vi "Read.vi"(0 "Setpoint Array":waveform(dbl)[](array[waveform]), 7 "error in (no error)":errorcluster, 14 "Process_REF":string="Temperature", 15 "physical channels":tag, 17 "Abort":bool) -> (20 "Temperature Graph":waveform(dbl)[](graph), 21 "Thermocouple 1":dbl, 22 "Thermocouple 2":dbl, 23 "Thermocouple 3":dbl, 24 "Thermocouple 4":dbl, 25 "Thermocouple 5":dbl, 27 "error out":errorcluster)   [LabVIEW 2018]
uses:
  <vilib>/DAQmx/read.llb/DAQmx Read (Analog 1D DBL NChan 1Samp).vi
  <vilib>/DAQmx/create/channels.llb/DAQmx Create Channel (AI-Temperature-Thermocouple).vi
  <vilib>/DAQmx/miscellaneous.llb/DAQmx Fill In Error Info.vi
  <vilib>/Waveform/WDTOps.llb/WDT Append Waveforms DBL.vi
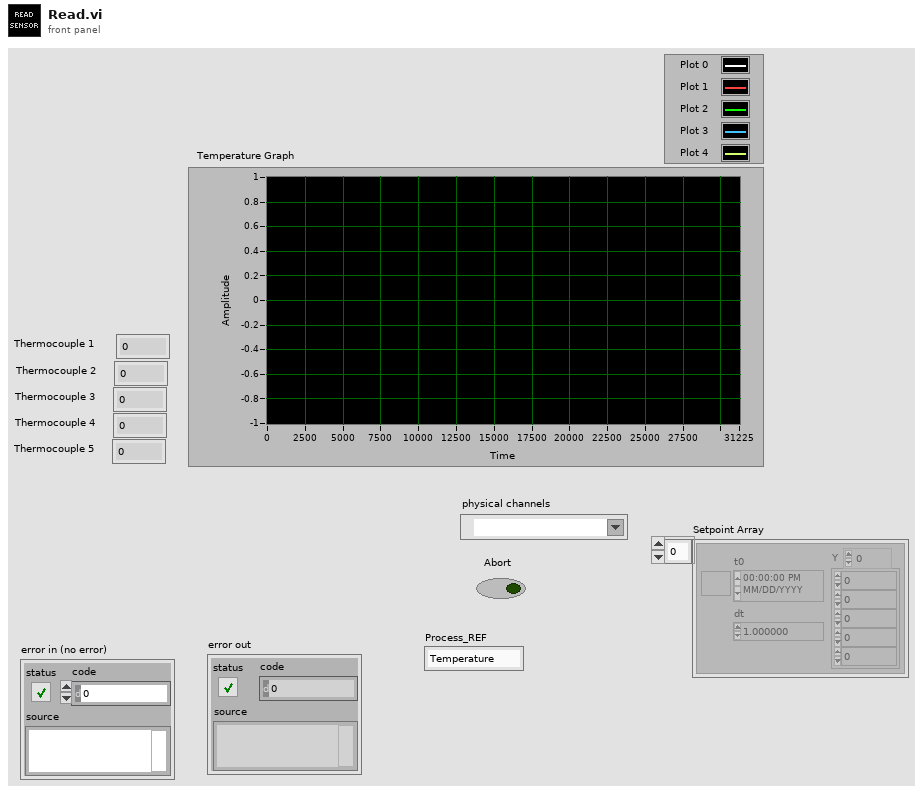
[diagram p1: front panel]
types:
  T1 = cluster{"data[0]":dbl, "data[1]":dbl, "data[2]":dbl, "data[3]":dbl, "data[4]":dbl}
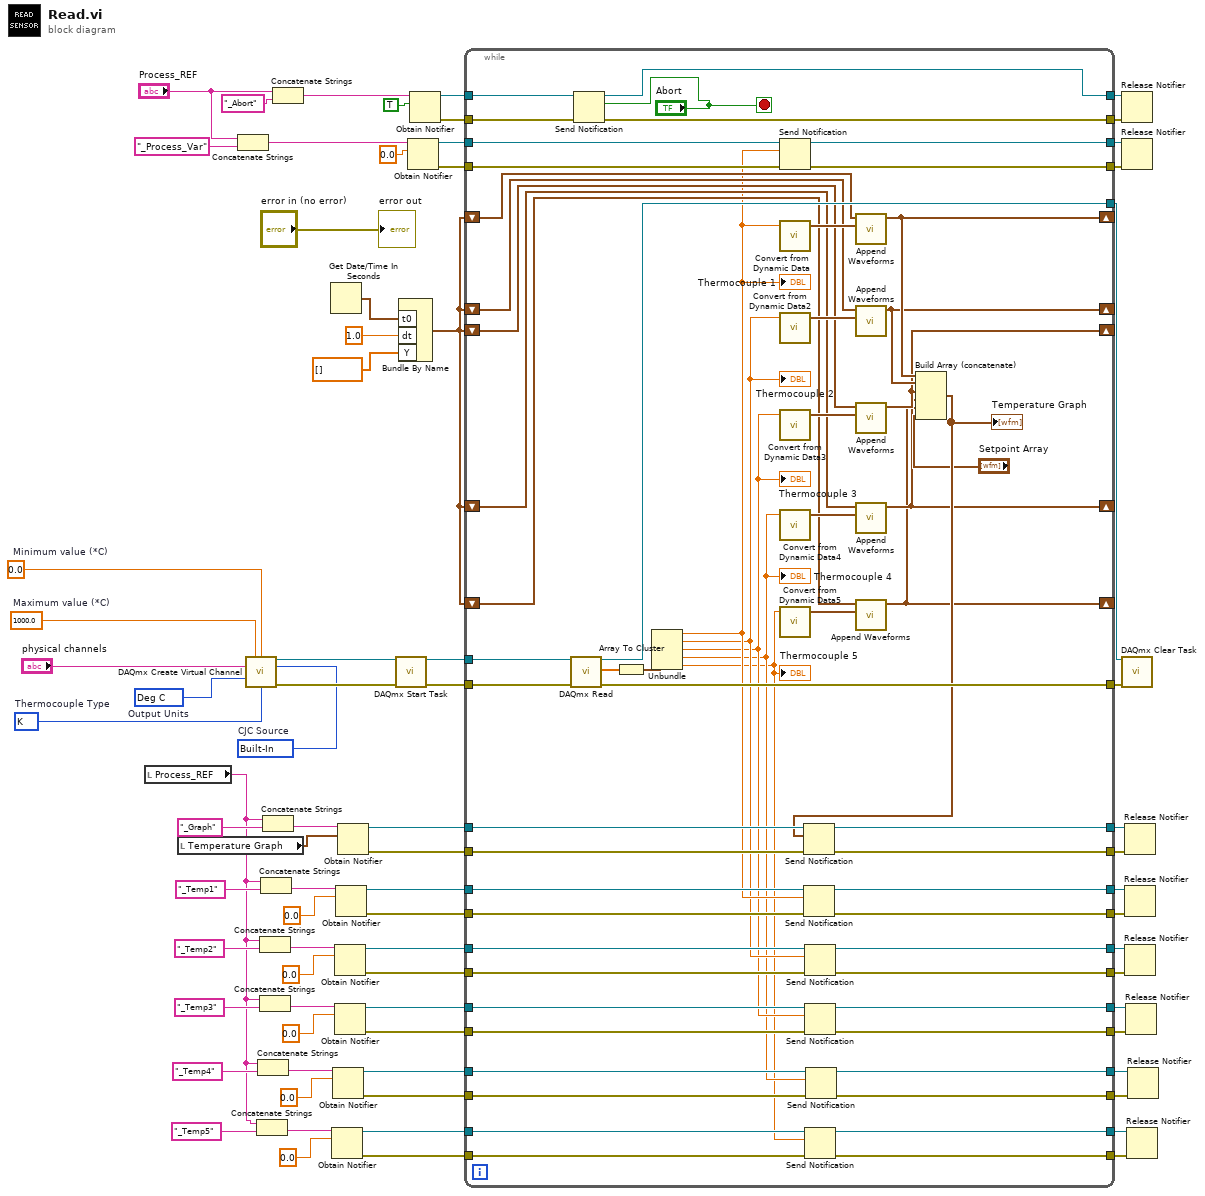
[diagram p0: block diagram]
diagram:
  w70 = 10143 items=["Deg C"=10143, "Deg F"=10144, "Kelvins"=10325, "Deg R"=10145, "From Custom Scale"=10065]  # Output Units
  w73 = 10073 items=["J"=10072, "K"=10073, "N"=10077, "R"=10082, "S"=10085, "T"=10086, "B"=10047, "E"=10055]  # Thermocouple Type
  w71 = 1000.0  # Maximum value (*C)
  w72 = 0.0  # Minimum value (*C)
  w69 = 10200 items=["Built-In"=10200, "Constant Value"=10116, "Channel"=10113]  # CJC Source
  n1 = local read "Process_REF"() -> (w1:string)
  n2 = local read "Temperature Graph"() -> (w17:waveform(dbl)[])
  n3 = Concatenate Strings("Process_REF", "_Process_Var" ("name (unnamed)")) -> (w50:string)
  n4 = call-poly <vilib>:"DAQmx Create Virtual Channel.vi"("maximum value"=w71, "minimum value"=w72, "physical channels"="physical channels", "cjc source"=w69, "units"=w70, "thermocouple type"=w73) -> ("task out"=w75:refnum<k21>, "error out"=w74:errorcluster)  [unwired: 8 in]
  n5 = Concatenate Strings(w1, "_Temp5") -> (w26:string)
  n6 = Concatenate Strings(w1, "_Temp4") -> (w29:string)
  n7 = Concatenate Strings(w1, "_Temp2") -> (w35:string)
  n8 = Concatenate Strings(w1, "_Temp3") -> (w32:string)
  n9 = Concatenate Strings(w1, "_Temp1") -> (w42:string)
  n10 = Concatenate Strings(w1, "_Graph") -> (w19:string)
  n11 = Concatenate Strings("Process_REF", "_Abort") -> (w49:string)
  n12 = Get Date/Time In Seconds() -> (seconds since 1Jan1904=w47:timestamp)
  n13 = Obtain Notifier(name (unnamed)=w26, notification data type=0.0) -> (notifier out=w21:refnum<notifier>, error out=w13:errorcluster)  [unwired: 2 in, 1 out]
  n14 = Obtain Notifier(name (unnamed)=w29, notification data type=0.0) -> (notifier out=w22:refnum<notifier>, error out=w12:errorcluster)  [unwired: 2 in, 1 out]
  n15 = Obtain Notifier(name (unnamed)=w35, notification data type=0.0) -> (notifier out=w24:refnum<notifier>, error out=w15:errorcluster)  [unwired: 2 in, 1 out]
  n16 = Obtain Notifier(name (unnamed)=w32, notification data type=0.0) -> (notifier out=w23:refnum<notifier>, error out=w14:errorcluster)  [unwired: 2 in, 1 out]
  n17 = Obtain Notifier(name (unnamed)=w42, notification data type=0.0) -> (notifier out=w40:refnum<notifier>, error out=w38:errorcluster)  [unwired: 2 in, 1 out]
  n18 = Obtain Notifier(name (unnamed)=w19, notification data type=w17) -> (notifier out=w18:refnum<notifier>, error out=w16:errorcluster)  [unwired: 2 in, 1 out]
  n19 = call <vilib>:"DAQmx Start Task.vi"("task/channels in"=w75, "error in"=w74) -> ("task out"=w67:refnum<k21>, "error out"=w66:errorcluster)  [unwired: 12 in]
  n20 = Bundle By Name("t0"=w47, "dt"=1.0, "Y"=dbl[] []) -> (w44:waveform(dbl))  [unwired: 1 in]
  n21 = Obtain Notifier(name (unnamed)=w50, notification data type=0.0) -> (notifier out=w63:refnum<notifier>, error out=w62:errorcluster)  [unwired: 2 in, 1 out]
  n22 = Obtain Notifier(name (unnamed)=w49, notification data type=TRUE) -> (notifier out=w58:refnum<notifier>, error out=w57:errorcluster)  [unwired: 2 in, 1 out]
  n23 = while {
    tunnel: w67 -> [w136]
    tunnel: w66 -> [w135]
    tunnel: [w134] -> w65
    tunnel: [w133] -> w64
    tunnel: w63 -> [w132]
    tunnel: w62 -> [w131]
    tunnel: [w130] -> w61
    tunnel: [w129] -> w60
    tunnel: w58 -> [w118]
    tunnel: w57 -> [w115]
    tunnel: [w117] -> w56
    tunnel: [w116] -> w55
    shift-right: [w80] -> _
    shift-left: w44 -> [w123]
    shift-right: [w79] -> _
    shift-left: w44 -> [w122]
    shift-right: [w78] -> _
    shift-left: w44 -> [w121]
    shift-right: [w77] -> _
    shift-left: w44 -> [w120]
    shift-right: [w76] -> _
    shift-left: w44 -> [w119]
    tunnel: [w110] -> w39
    tunnel: w40 -> [w111]
    tunnel: w38 -> [w109]
    tunnel: [w108] -> w37
    tunnel: w24 -> [w105]
    tunnel: w23 -> [w106]
    tunnel: w22 -> [w104]
    tunnel: w21 -> [w107]
    tunnel: [w103] -> w5
    tunnel: w18 -> [w102]
    tunnel: w16 -> [w101]
    tunnel: w15 -> [w100]
    tunnel: w14 -> [w99]
    tunnel: w13 -> [w98]
    tunnel: w12 -> [w97]
    tunnel: [w95] -> w2
    tunnel: [w94] -> w3
    tunnel: [w93] -> w4
    tunnel: [w92] -> w6
    tunnel: [w91] -> w7
    tunnel: [w90] -> w9
    tunnel: [w89] -> w8
    tunnel: [w88] -> w11
    tunnel: [w87] -> w10
    stop <- "Abort" stop-if-true
    n24 = call-poly <vilib>:"DAQmx Read.vi"("task/channels in"=w136, "error in"=w135) -> ("task out"=w134:refnum<k21>, "data"=w113:dbl[], "error out"=w133:errorcluster)  [unwired: 11 in]
    n25 = Send Notification(notification="Abort", notifier=w118, error in (no error)=w115) -> (notifier out=w117:refnum<notifier>, error out=w116:errorcluster)
    n26 = Array To Cluster(array=w113) -> (cluster=w112:T1)
    n27 = Unbundle(w112) -> ("data[0]"=w86:dbl, "data[1]"=w85:dbl, "data[2]"=w84:dbl, "data[3]"=w83:dbl, "data[4]"=w82:dbl)
    "Thermocouple 1" <- w86
    "Thermocouple 2" <- w85
    "Thermocouple 3" <- w84
    "Thermocouple 4" <- w83
    "Thermocouple 5" <- w82
    n28 = Send Notification(notification=w86, notifier=w132, error in (no error)=w131) -> (notifier out=w130:refnum<notifier>, error out=w129:errorcluster)
    n29 = call "Convert from Dynamic Data"("Dynamic Data Type"=w86) -> ("Waveform"=w128:waveform(dbl))  [unwired: 3 in]
    n30 = call "Convert from Dynamic Data2"("Dynamic Data Type"=w85) -> ("Waveform"=w127:waveform(dbl))  [unwired: 3 in]
    n31 = call "Convert from Dynamic Data3"("Dynamic Data Type"=w84) -> ("Waveform"=w126:waveform(dbl))  [unwired: 3 in]
    n32 = call "Convert from Dynamic Data4"("Dynamic Data Type"=w83) -> ("Waveform"=w125:waveform(dbl))  [unwired: 3 in]
    n33 = call "Convert from Dynamic Data5"("Dynamic Data Type"=w82) -> ("Waveform"=w124:waveform(dbl))  [unwired: 3 in]
    n34 = Send Notification(notification=w86, notifier=w111, error in (no error)=w109) -> (notifier out=w110:refnum<notifier>, error out=w108:errorcluster)
    n35 = Send Notification(notification=w85, notifier=w105, error in (no error)=w100) -> (notifier out=w103:refnum<notifier>, error out=w93:errorcluster)
    n36 = Send Notification(notification=w84, notifier=w106, error in (no error)=w99) -> (notifier out=w91:refnum<notifier>, error out=w92:errorcluster)
    n37 = Send Notification(notification=w82, notifier=w107, error in (no error)=w98) -> (notifier out=w88:refnum<notifier>, error out=w87:errorcluster)
    n38 = Send Notification(notification=w83, notifier=w104, error in (no error)=w97) -> (notifier out=w90:refnum<notifier>, error out=w89:errorcluster)
    n39 = call-poly <vilib>:"Append Waveforms.vi"("waveform B"=w128, "waveform A"=w123) -> ("waveform out"=w80:waveform(dbl))  [unwired: 8 in, 1 out]
    n40 = call-poly <vilib>:"Append Waveforms.vi"("waveform B"=w127, "waveform A"=w122) -> ("waveform out"=w79:waveform(dbl))  [unwired: 8 in, 1 out]
    n41 = call-poly <vilib>:"Append Waveforms.vi"("waveform B"=w126, "waveform A"=w121) -> ("waveform out"=w78:waveform(dbl))  [unwired: 8 in, 1 out]
    n42 = call-poly <vilib>:"Append Waveforms.vi"("waveform B"=w125, "waveform A"=w120) -> ("waveform out"=w77:waveform(dbl))  [unwired: 8 in, 1 out]
    n43 = call-poly <vilib>:"Append Waveforms.vi"("waveform B"=w124, "waveform A"=w119) -> ("waveform out"=w76:waveform(dbl))  [unwired: 8 in, 1 out]
    n44 = Build Array (concatenate)(w80, w79, w78, w77, w76, "Setpoint Array") -> (w96:waveform(dbl)[])
    "Temperature Graph" <- w96
    n45 = Send Notification(notification=w96, notifier=w102, error in (no error)=w101) -> (notifier out=w95:refnum<notifier>, error out=w94:errorcluster)
  }
  n46 = Release Notifier(notifier=w56, error in (no error)=w55) -> ()  [unwired: 1 in, 3 out]
  n47 = Release Notifier(notifier=w61, error in (no error)=w60) -> ()  [unwired: 1 in, 3 out]
  n48 = call <vilib>:"DAQmx Clear Task.vi"("task in"=w65, "error in"=w64) -> ()  [unwired: 13 in, 1 out]
  n49 = Release Notifier(notifier=w2, error in (no error)=w3) -> ()  [unwired: 1 in, 3 out]
  n50 = Release Notifier(notifier=w39, error in (no error)=w37) -> ()  [unwired: 1 in, 3 out]
  n51 = Release Notifier(notifier=w5, error in (no error)=w4) -> ()  [unwired: 1 in, 3 out]
  n52 = Release Notifier(notifier=w7, error in (no error)=w6) -> ()  [unwired: 1 in, 3 out]
  n53 = Release Notifier(notifier=w11, error in (no error)=w10) -> ()  [unwired: 1 in, 3 out]
  n54 = Release Notifier(notifier=w9, error in (no error)=w8) -> ()  [unwired: 1 in, 3 out]
  "error out" <- "error in (no error)"
